vi "曲线对齐-多曲线.vi"() -> ()   [LabVIEW 2015]
uses:
  <vilib>/Utility/miscctls.llb/LVCursorListTypeDef.ctl
  <vilib>/gmath/NI_Gmath.lvlib
panel:
  in  "参考曲线":u16(ring) items=["数据1", "数据2"]
  in  "编辑曲线":u16(ring) items=["数据1", "数据2"]
  in  "重采样间隔":dbl=0.1 min=1e-06 format="%.3fs"
  in  "取消修改":bool
  in  "当前编辑曲线":T1
  in  "确认修改":bool
  in  "功能选择":T2
  in  "加载数据":bool
  out "曲线对齐":cluster{"理论时间":dbl[], "力":dbl[]}[](graph)
  in  "测量曲线路径":path=path "D:/曲线处理/数据源.csv" caption="数据源"
  in  "Enqueue Element":bool caption="元素入队列"
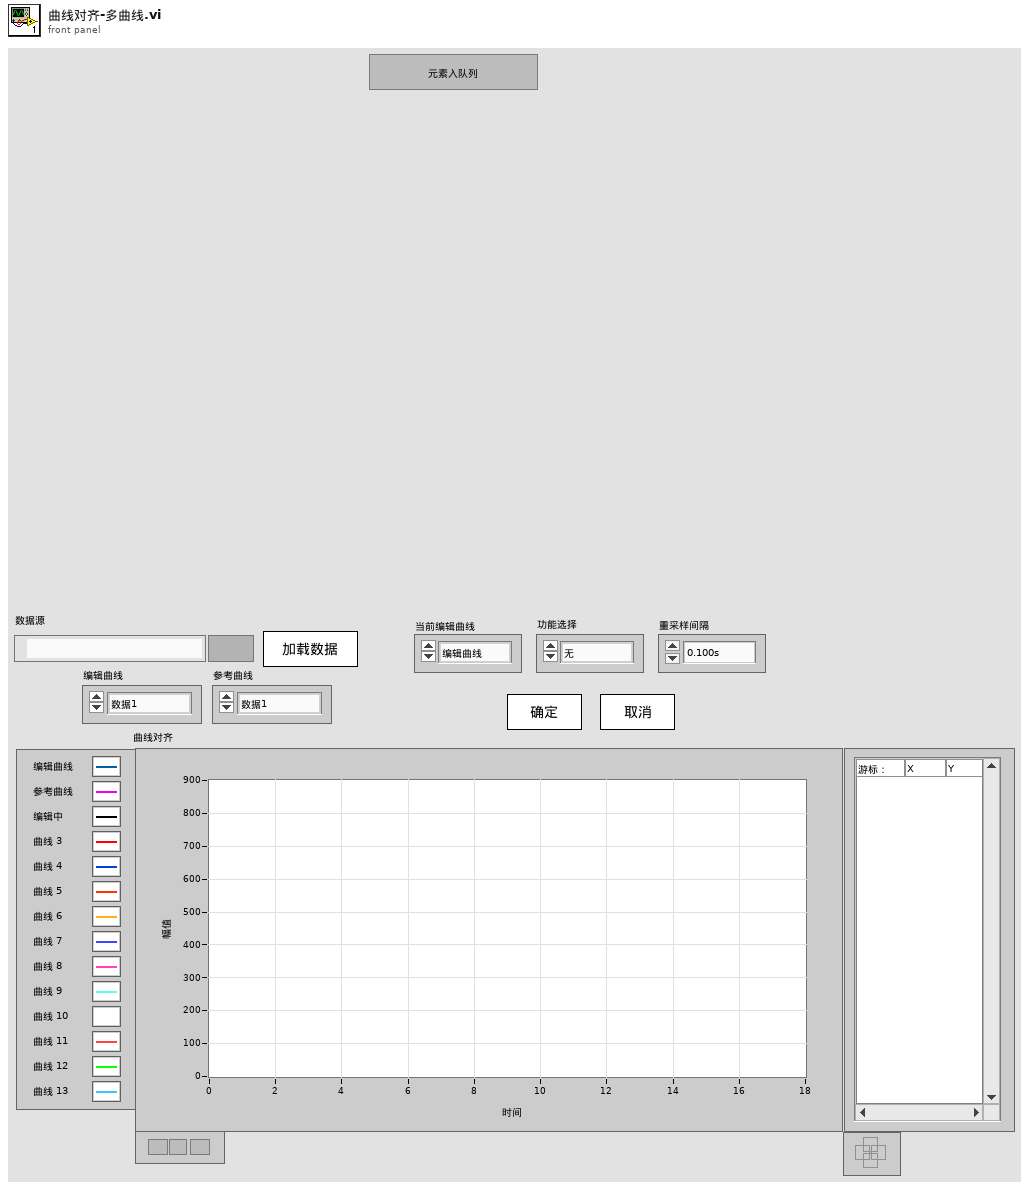
[diagram p1: front panel]
types:
  T1 = typedef "曲线选择.ctl" = enum16{"编辑曲线", "参考曲线"}
  T2 = typedef "功能选择.ctl" = enum16{"无", "缩放曲线", "剪裁曲线", "对齐曲线", "初始值置0", "重采样", "曲线平滑"}
  T3 = typedef "曲线定义.ctl" = enum16{"编辑曲线", "参考曲线", "编辑中曲线"}
  T4 = typedef "LVCursorListTypeDef.ctl" = cluster{"Name":string, "Color":u32, "Style":u8, "Point Style":u8, "Name Visible":bool, "Allow Drag":bool, "Cursor Mode":u32, "Plot":i32, "Index":i32, "Position":cluster{"X":dbl, "Y":dbl}, "X Scale":u32, "Y Scale":u32, "Watch Plots":i32[], "Watch All Plots":bool, "Plot Area":i32, "Label Offset":cluster{"X":dbl, "Y":dbl}}[]
  T5 = cluster{"Name":string, "Color":u32, "Style":u8, "Point Style":u8, "Name Visible":bool, "Allow Drag":bool, "Cursor Mode":u32, "Plot":i32, "Index":i32, "Position":cluster{"X":dbl, "Y":dbl}, "X Scale":u32, "Y Scale":u32, "Watch Plots":i32[], "Watch All Plots":bool, "Plot Area":i32, "Label Offset":cluster{"X":dbl, "Y":dbl}}
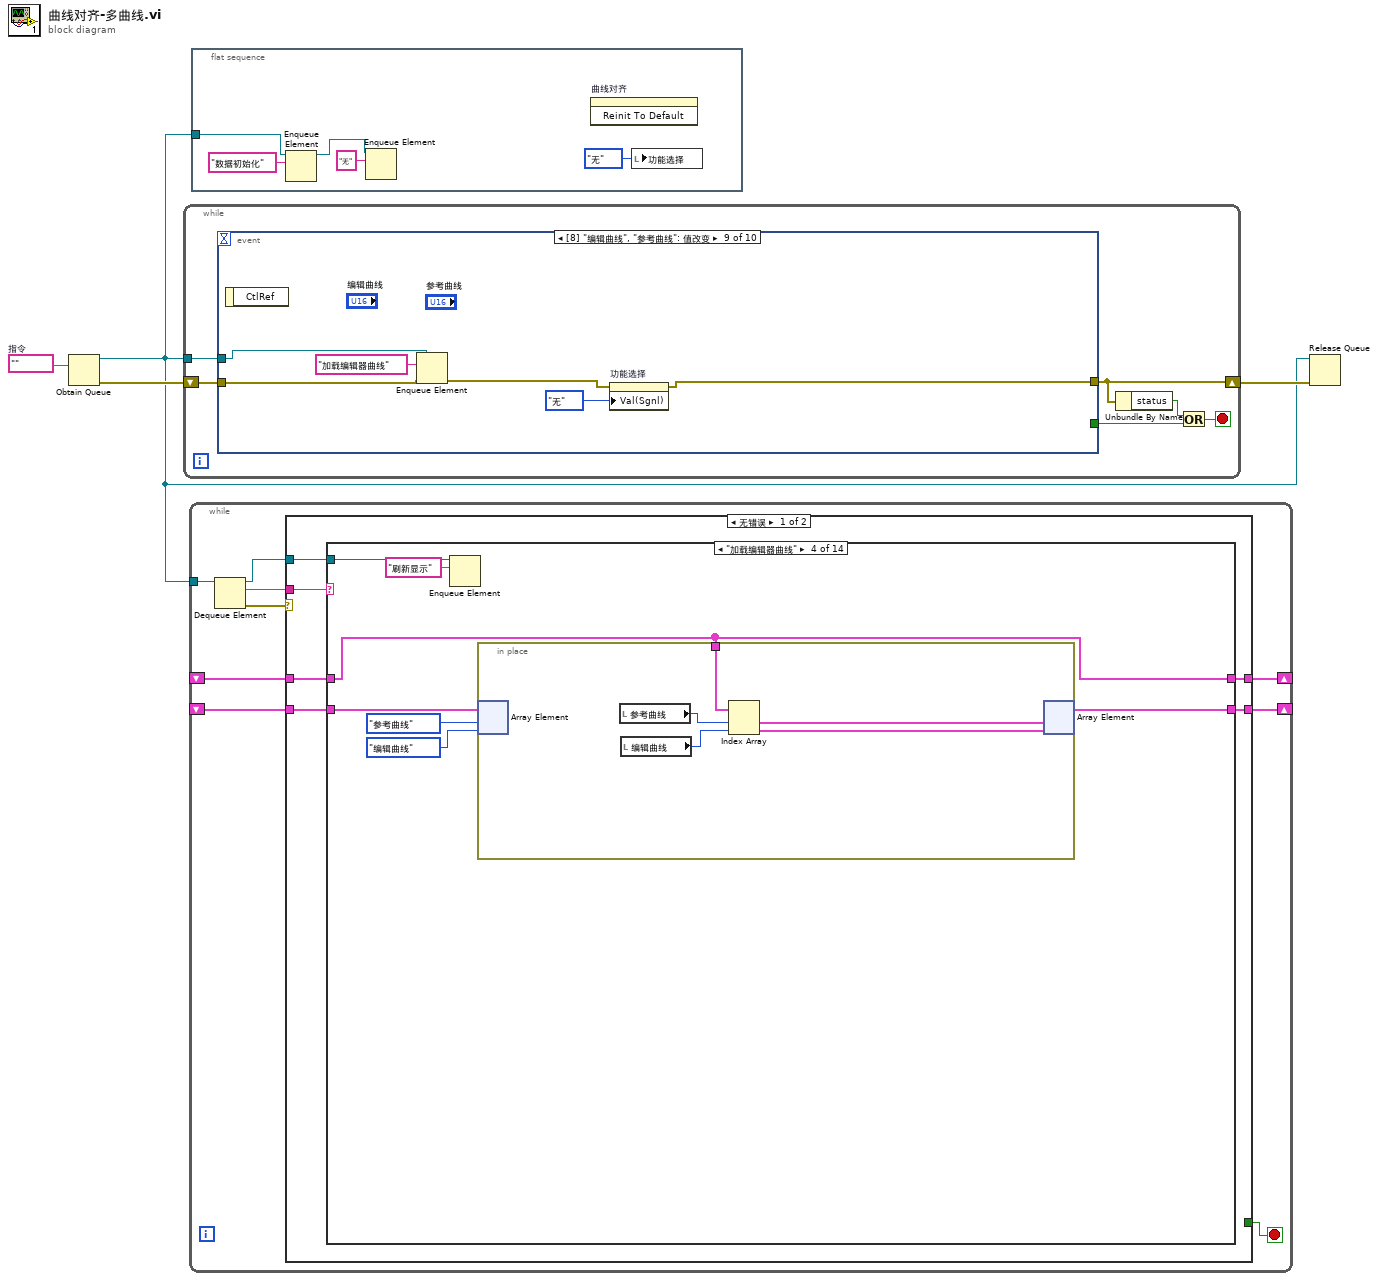
[diagram p0: block diagram]
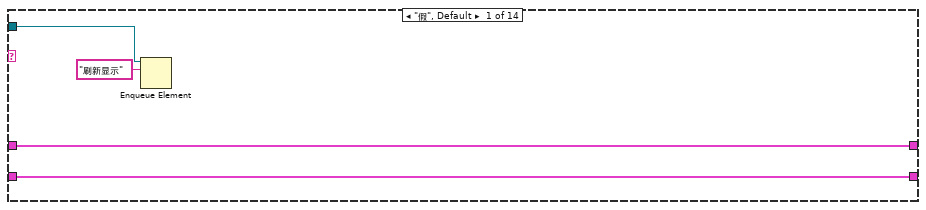
[diagram p2: hidden frame]
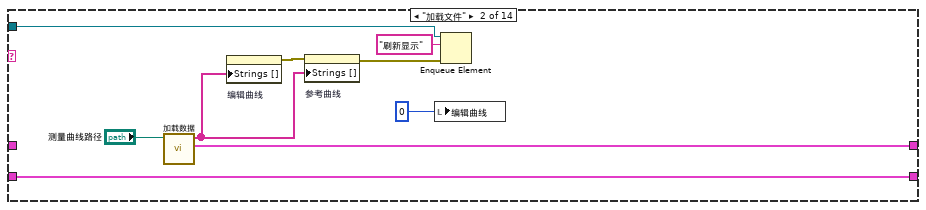
[diagram p3: hidden frame]
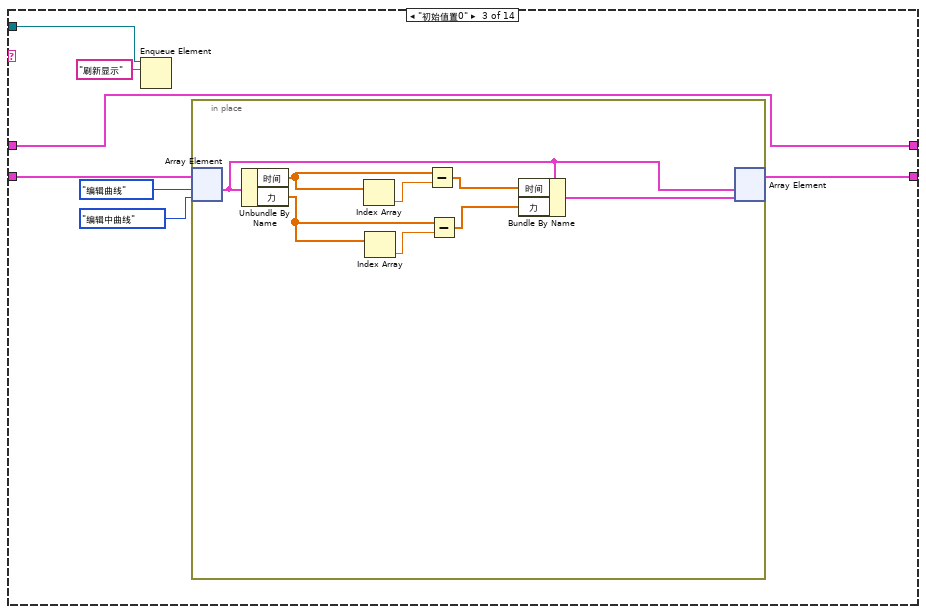
[diagram p4: hidden frame]
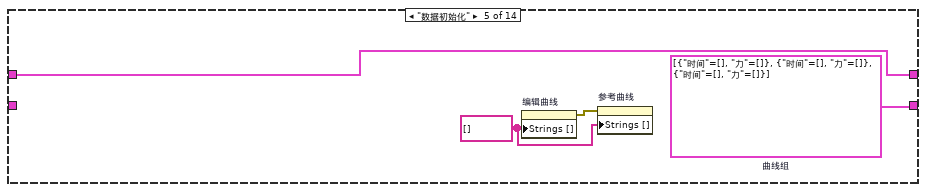
[diagram p5: hidden frame]
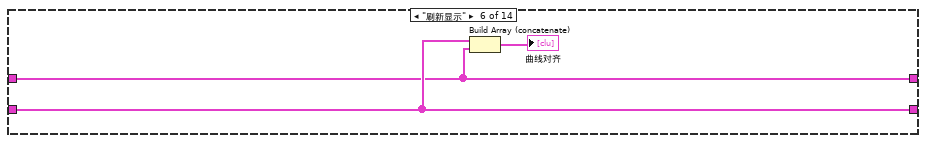
[diagram p6: hidden frame]
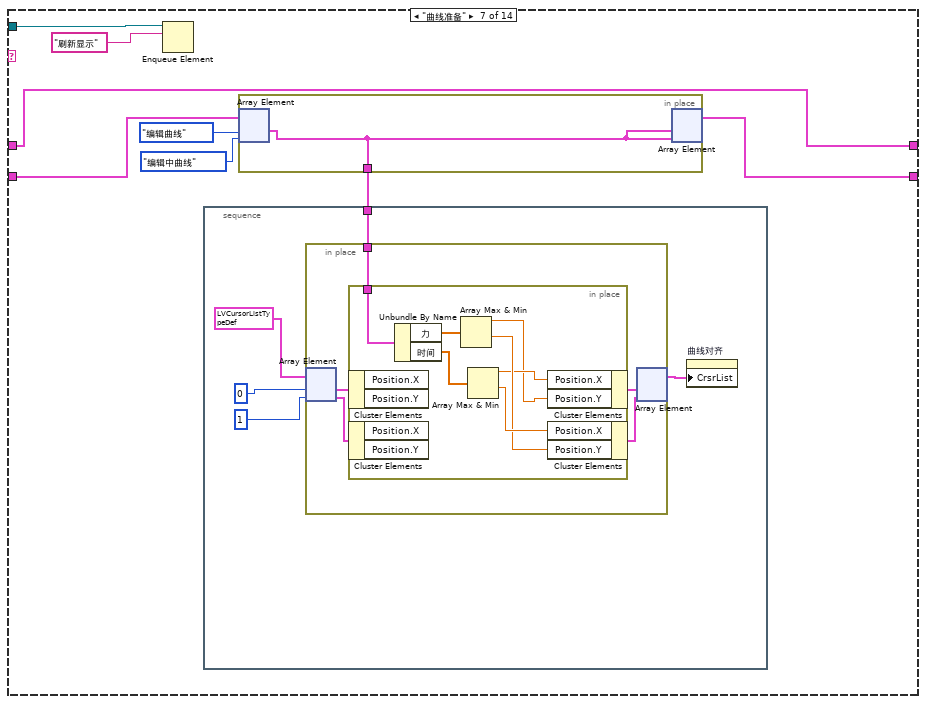
[diagram p7: hidden frame]
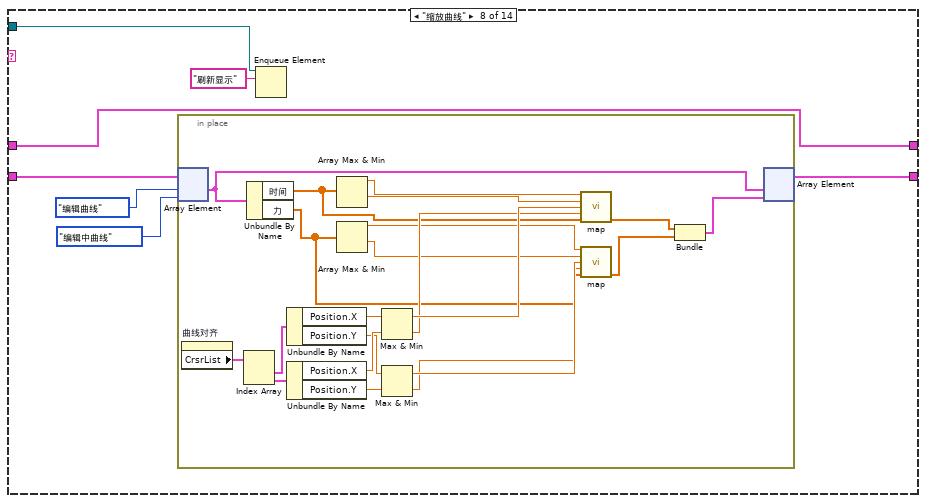
[diagram p8: hidden frame]
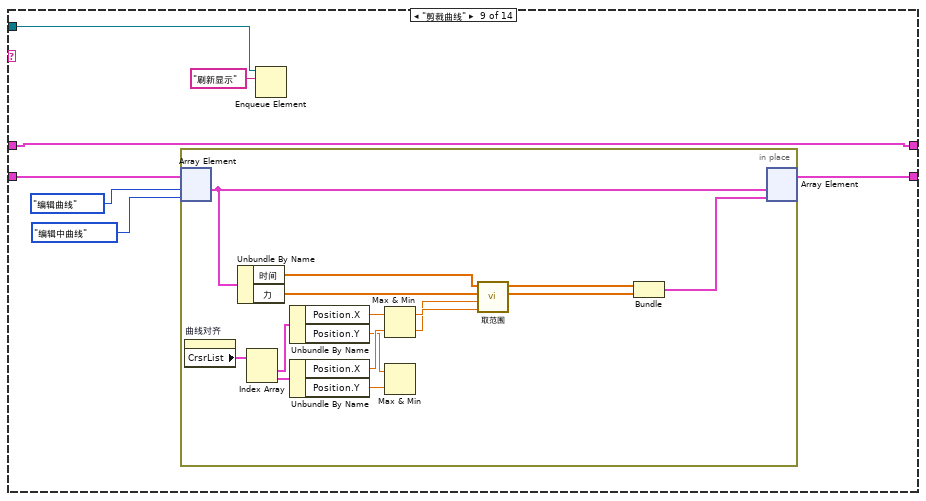
[diagram p9: hidden frame]
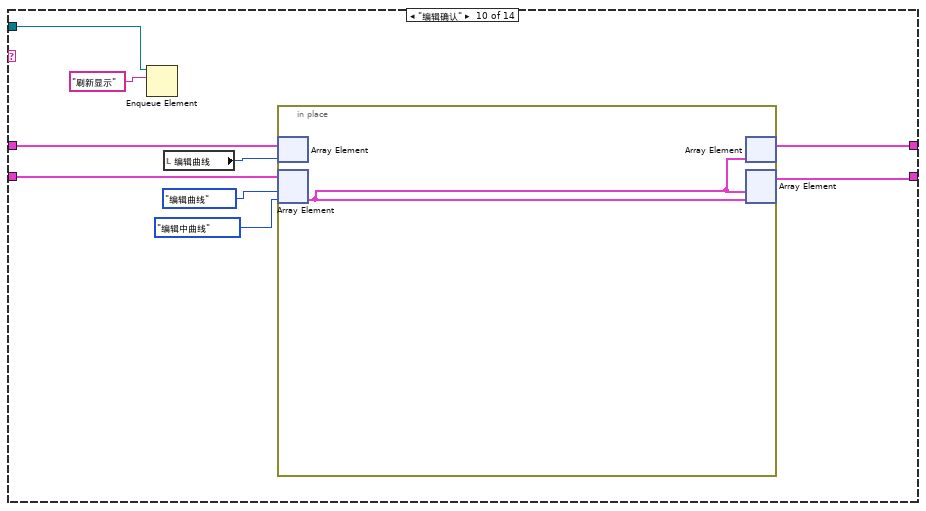
[diagram p10: hidden frame]
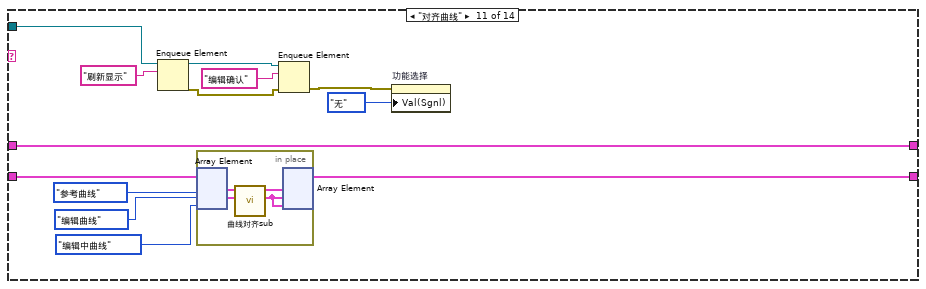
[diagram p11: hidden frame]
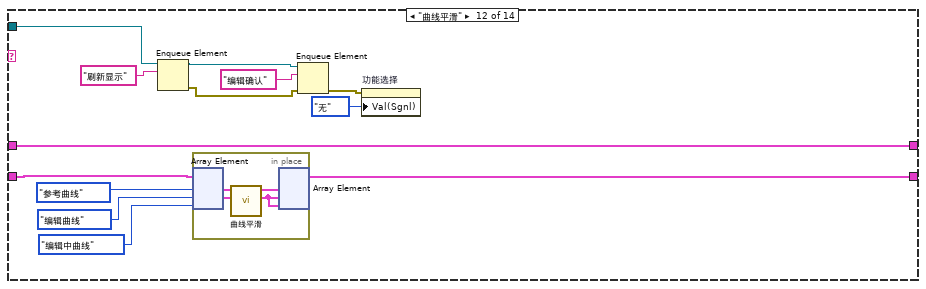
[diagram p12: hidden frame]
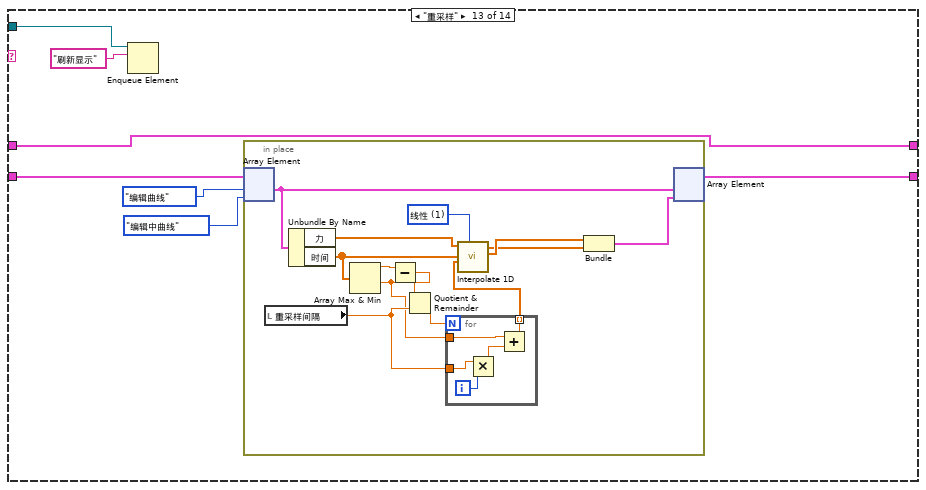
[diagram p13: hidden frame]
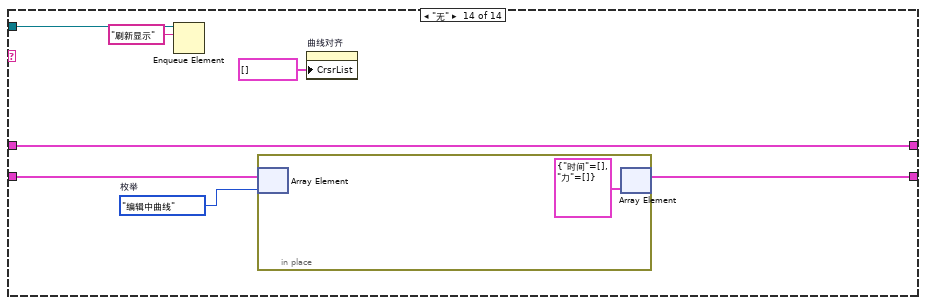
[diagram p14: hidden frame]
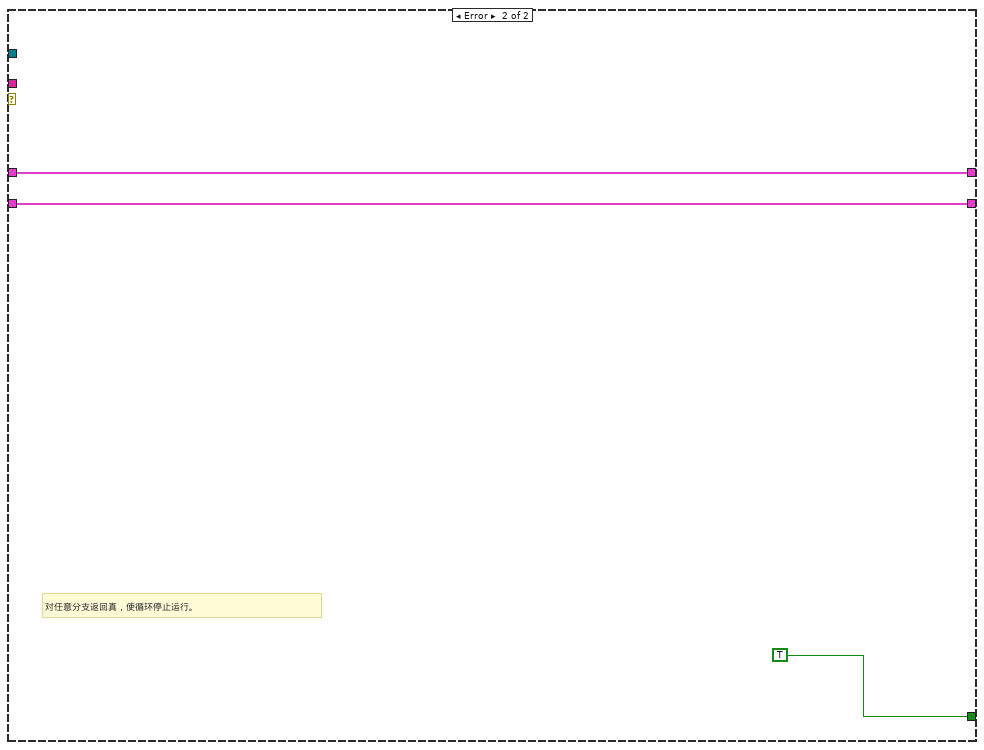
[diagram p15: hidden frame]
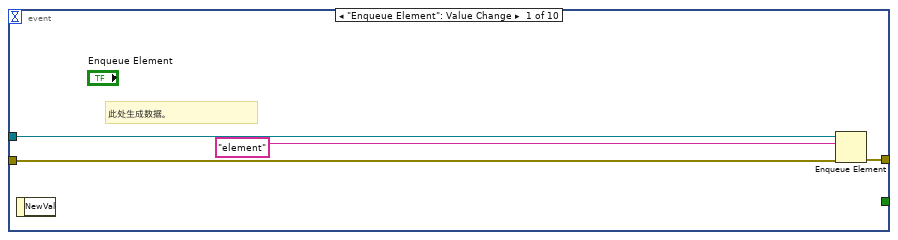
[diagram p16: hidden frame]
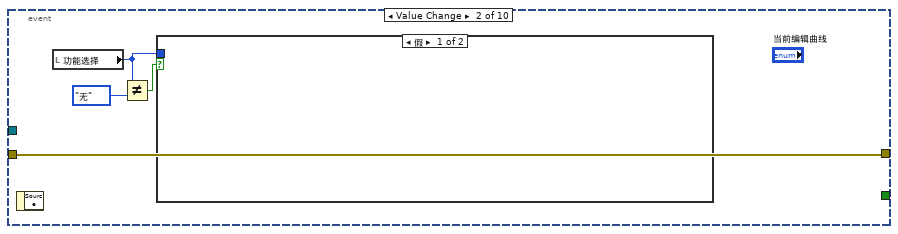
[diagram p17: hidden frame]
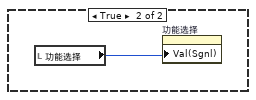
[diagram p18: hidden frame]
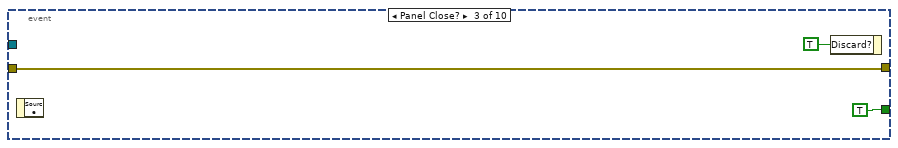
[diagram p19: hidden frame]
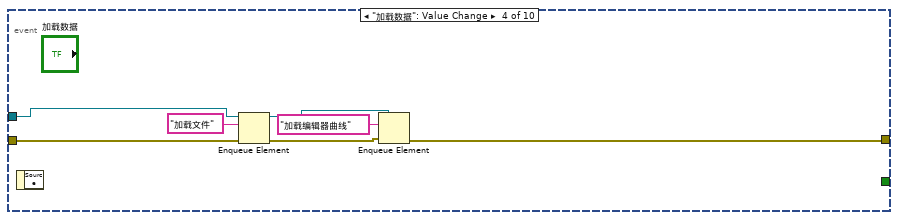
[diagram p20: hidden frame]
diagram:
  w4 = ""  # 指令
  n1 = Obtain Queue(element data type=w4) -> (queue out=w1:refnum<queue>, error out=w2:errorcluster)  [unwired: 4 in, 1 out]
  n2 = while {
    shift-right: [w6] -> w3
    shift-left: w2 -> [w9]
    tunnel: w1 -> [w10]
    stop <- w7 stop-if-true
    n3 = event shown="[8] \"编辑曲线\", \"参考曲线\": 值改变" {
      selector: _ -> [_ _ _ _ _ _ _ _ _ _]
      dyn-events: _ -> [_ _ _ _ _ _ _ _ _ _]
      timeout: _ -> [_ _ _ _ _ _ _ _ _ _]
      tunnel: w10 -> [w14 _ _ w27 w33 _ w43 w49 w70 w72]
      tunnel: w9 -> [w13 w18 w22 w26 w34 w38 w44 w51 w69 w74]
      tunnel: [w12 w18 w22 w23 w34 w37 w44 w51 w66 w74] -> w6
      tunnel: [_ _ TRUE ("stop") _ _ _ _ _ _ _] -> w8
      event "Enqueue Element": Value Change {
        # "此处生成数据。"
        n4 = event-data() -> ()  [unwired: 1 in, 1 out]
        n5 = Enqueue Element(queue=w14, element="element", error in (no error)=w13) -> (error out=w12:errorcluster)  [unwired: 1 in, 2 out]
      }
      event Value Change {
        n6 = event-data() -> ()  [unwired: 1 in, 1 out]
        n7 = local read "功能选择"() -> (w15:T2)
        n8 = Not Equal?(x=w15, y=功能选择."无") -> (x != y?=w17:bool)
        n9 = case shown="假" w17 {
          tunnel: w15 -> [_ _]
          frame False {
          }
          frame True {
            n10 = local read "功能选择"() -> (w19:T2)
            n11 = property on="功能选择" class="Enum (严格)"("Val(Sgnl)"=w19) -> ()  [unwired: 2 in, 2 out]
          }
        }
      }
      event Panel Close? {
        n12 = event-data() -> ()  [unwired: 1 in, 1 out]
        n13 = event-data("Discard?"=TRUE ("放弃？")) -> ()  [unwired: 1 in, 1 out]
      }
      event "加载数据": Value Change {
        n14 = event-data() -> ()  [unwired: 1 in, 1 out]
        n15 = Enqueue Element(queue=w27, element="加载文件" ("元素"), error in (no error)=w26) -> (queue out=w24:refnum<queue>, error out=w25:errorcluster)  [unwired: 1 in, 1 out]
        n16 = Enqueue Element(queue=w24, element="加载编辑器曲线" ("元素"), error in (no error)=w25) -> (error out=w23:errorcluster)  [unwired: 1 in, 2 out]
      }
      event "确认修改": Value Change {
        n17 = event-data() -> ()  [unwired: 1 in, 1 out]
        n18 = local read "功能选择"() -> (w32:T2)
        n19 = Not Equal?(x=w32, y=功能选择."无") -> (x != y?=w31:bool)
        n20 = case shown="真" w31 {
          tunnel: w33 -> [_ w35]
          frame False {
          }
          frame True {
            n21 = Enqueue Element(queue=w35, element="编辑确认" ("元素")) -> ()  [unwired: 2 in, 3 out]
          }
        }
      }
      event "取消修改": Value Change {
        n22 = event-data() -> ()  [unwired: 1 in, 1 out]
        n23 = property on="功能选择" class="Enum (严格)"(error in=w38, "Val(Sgnl)"=功能选择."无" ("值(信号)")) -> (error out=w37:errorcluster)  [unwired: 1 in, 1 out]
      }
      event "重采样间隔": Value Change {
        n24 = event-data() -> ()  [unwired: 1 in, 1 out]
        n25 = local read "功能选择"() -> (w41:T2)
        n26 = Equal?(x=w41, y=功能选择."重采样") -> (x = y?=w42:bool)
        n27 = case shown="真" w42 {
          tunnel: w43 -> [_ w45]
          frame False {
          }
          frame True {
            n28 = Enqueue Element(queue=w45, element="重采样" ("元素")) -> ()  [unwired: 2 in, 3 out]
          }
        }
      }
      event Value Change {
        n29 = event-data() -> ("NewVal"=w50:T2)  [unwired: 1 in]
        n30 = Enqueue Element(queue=w49, element="无" ("元素")) -> (queue out=w48:refnum<queue>)  [unwired: 2 in, 2 out]
        n31 = case shown="\"初始值置0\"" w50 {
          tunnel: w48 -> [w52 w55 w56 w58 w60 w63 w64]
          frame "缩放曲线", Default {
            n32 = Enqueue Element(queue=w52, element="曲线准备" ("元素")) -> ()  [unwired: 2 in, 3 out]
          }
          frame "无" {
            n33 = Enqueue Element(queue=w55, element="无" ("元素")) -> ()  [unwired: 2 in, 3 out]
          }
          frame "剪裁曲线" {
            n34 = Enqueue Element(queue=w56, element="曲线准备" ("元素")) -> ()  [unwired: 2 in, 3 out]
          }
          frame "对齐曲线" {
            n35 = Enqueue Element(queue=w58, element="对齐曲线" ("元素")) -> ()  [unwired: 2 in, 3 out]
          }
          frame "初始值置0" {
            n36 = Enqueue Element(queue=w60, element="初始值置0" ("元素")) -> ()  [unwired: 2 in, 3 out]
          }
          frame "重采样" {
            n37 = Enqueue Element(queue=w63, element="重采样" ("元素")) -> ()  [unwired: 2 in, 3 out]
          }
          frame "曲线平滑" {
            n38 = Enqueue Element(queue=w64, element="曲线平滑" ("元素")) -> ()  [unwired: 2 in, 3 out]
          }
        }
      }
      event "编辑曲线", "参考曲线": Value Change {
        n39 = event-data() -> ()  [unwired: 1 in, 1 out]
        n40 = Enqueue Element(queue=w70, element="加载编辑器曲线" ("元素"), error in (no error)=w69) -> (error out=w67:errorcluster)  [unwired: 1 in, 2 out]
        n41 = property on="功能选择" class="Enum (严格)"(error in=w67, "Val(Sgnl)"=功能选择."无" ("功能选择")) -> (error out=w66:errorcluster)  [unwired: 1 in, 1 out]
      }
      event "曲线对齐": Cursor Move {
        n42 = event-data() -> ()  [unwired: 1 in, 8 out]
        n43 = local read "功能选择"() -> (w73:T2)
        n44 = case shown="\"无\", 默认" w73 {
          tunnel: w72 -> [_ w75 w77]
          frame "无", Default {
          }
          frame "缩放曲线" {
            n45 = Enqueue Element(queue=w75, element="缩放曲线" ("元素")) -> ()  [unwired: 2 in, 3 out]
          }
          frame "剪裁曲线" {
            n46 = Enqueue Element(queue=w77, element="剪裁曲线" ("元素")) -> ()  [unwired: 2 in, 3 out]
          }
        }
      }
    }
    n47 = Unbundle By Name(w6) -> ("status"=w5:bool)
    n48 = Or(x=w5, y=w8) -> (x .or. y?=w7:bool)
  }
  n49 = while {
    tunnel: w1 -> [w82]
    shift-right: [w84] -> _
    shift-left: _ -> [w83]
    shift-right: [w80] -> _
    shift-left: _ -> [w79]
    stop <- w85 stop-if-true
    n50 = Dequeue Element(queue=w82) -> (queue out=w81:refnum<queue>, element=w86:string, error out=w87:errorcluster)  [unwired: 2 in, 1 out]
    n51 = case shown="无错误" w87 {
      tunnel: w86 -> [w93 _]
      tunnel: [_ TRUE] -> w85
      tunnel: [w90 w295] -> w84
      tunnel: w83 -> [w92 w295]
      tunnel: w81 -> [w91 _]
      tunnel: [w89 w294] -> w80
      tunnel: w79 -> [w88 w294]
      frame No Error {
        n52 = case shown="\"加载编辑器曲线\"" w93 {
          tunnel: [w95 w104 w111 w125 w137 w140 w144 w170 w198 w222 w236 w252 w264 w287] -> w90
          tunnel: w92 -> [w95 w104 w110 w126 _ w140 w145 w171 w199 w223 w235 w253 w265 w288]
          tunnel: w91 -> [w96 w105 w112 w128 _ _ w147 w172 w200 w224 w238 w255 w266 w290]
          tunnel: [w94 w102 w107 w123 w136 w139 w141 w167 w195 w217 w231 w248 w261 w289] -> w89
          tunnel: w88 -> [w94 _ w107 w123 w136 w139 w141 w167 w195 w218 w231 w248 w261 w289]
          frame "假", Default {
            n53 = Enqueue Element(queue=w96, element="刷新显示" ("元素")) -> ()  [unwired: 2 in, 3 out]
          }
          frame "加载文件" {
            n54 = call "加载数据.vi"("数据路径"="测量曲线路径") -> ("数据"=w102:cluster{dbl[], dbl[]}[], "数据名称"=w100:string[])  [unwired: 9 in]
            n55 = property on="编辑曲线" class="Ring (严格)"("Strings []"=w100) -> (error out=w99:errorcluster)  [unwired: 2 in, 1 out]
            n56 = property on="参考曲线" class="Ring (严格)"(error in=w99, "Strings []"=w100) -> (error out=w98:errorcluster)  [unwired: 1 in, 1 out]
            n57 = local write "编辑曲线"(0) -> ()
            n58 = Enqueue Element(queue=w105, element="刷新显示" ("元素"), error in (no error)=w98) -> ()  [unwired: 1 in, 3 out]
          }
          frame "初始值置0" {
            n59 = Enqueue Element(queue=w112, element="刷新显示" ("元素")) -> ()  [unwired: 2 in, 3 out]
            n60 = in-place {
              n61 = in-place-array #1(w110, 曲线定义."编辑曲线", 曲线定义."编辑中曲线") -> (w115:cluster{"时间":dbl[], "力":dbl[]})  [unwired: 1 out]
              n62 = Unbundle By Name(w115) -> ("时间"=w121:dbl[], "力"=w119:dbl[])
              n63 = Index Array(array=w121) -> (element=w120:dbl)  [unwired: 1 in]
              n64 = Index Array(array=w119) -> (element=w118:dbl)  [unwired: 1 in]
              n65 = Subtract(x=w121, y=w120) -> (x-y=w117:dbl[])
              n66 = Subtract(x=w119, y=w118) -> (x-y=w116:dbl[])
              n67 = Bundle By Name(cluster=w115, "时间"=w117, "力"=w116) -> (w114:cluster{"时间":dbl[], "力":dbl[]})
              n68 = in-place-array #1(w115, w114) -> (w111:cluster{"时间":dbl[], "力":dbl[]}[])  [unwired: 2 out]
            }
          }
          frame "加载编辑器曲线" {
            n69 = Enqueue Element(queue=w128, element="刷新显示" ("元素")) -> ()  [unwired: 2 in, 3 out]
            n70 = in-place {
              in-place-border: w123 -> [w133]
              n71 = in-place-array #2(w126, 曲线定义."参考曲线", 曲线定义."编辑曲线") -> ()  [unwired: 2 out]
              n72 = local read "参考曲线"() -> (w129:u16)
              n73 = local read "编辑曲线"() -> (w130:u16)
              n74 = Index Array(array=w133, index #1=w129, index #2=w130) -> (element #1=w132:cluster{dbl[], dbl[]}, element #2=w131:cluster{dbl[], dbl[]})
              n75 = in-place-array #2(w132, w131) -> (w125:cluster{"时间":dbl[], "力":dbl[]}[])  [unwired: 2 out]
            }
          }
          frame "数据初始化" {
            w135 = string[] [] ("字符串[]")
            w137 = cluster{"时间":dbl[], "力":dbl[]}[] [{"时间"=[], "力"=[]}, {"时间"=[], "力"=[]}, {"时间"=[], "力"=[]}]  # 曲线组
            n76 = property on="编辑曲线" class="Ring (严格)"("Strings []"=w135) -> (error out=w134:errorcluster)  [unwired: 2 in, 1 out]
            n77 = property on="参考曲线" class="Ring (严格)"(error in=w134, "Strings []"=w135) -> ()  [unwired: 1 in, 2 out]
          }
          frame "刷新显示" {
            n78 = Build Array (concatenate)(w140, w139) -> (→"曲线对齐":cluster{"时间":dbl[], "力":dbl[]}[])
          }
          frame "曲线准备" {
            n79 = Enqueue Element(queue=w147, element="刷新显示" ("元素")) -> ()  [unwired: 2 in, 3 out]
            n80 = in-place {
              in-place-border: [w149] -> w146
              n81 = in-place-array #3(w145, 曲线定义."编辑曲线", 曲线定义."编辑中曲线") -> (w149:cluster{"时间":dbl[], "力":dbl[]})  [unwired: 1 out]
              n82 = in-place-array #3(w149, w149) -> (w144:cluster{"时间":dbl[], "力":dbl[]}[])  [unwired: 2 out]
            }
            n83 = stacked-sequence {
              tunnel: w146 -> [w150]
              frame #0 {
                n84 = in-place {
                  in-place-border: w150 -> [w155]
                  n85 = in-place-array #4(T4 [{"Name"="游标0", "Color"=16711680, "Style"=8, "Point Style"=13, "Name Visible"=FALSE, "Allow Drag"=TRUE, "Cursor Mode"=0, "Plot"=0, "Index"=0, "Position"={"X"=24.900169204737733, "Y"=876.3513513513514}, "X Scale"=0, "Y Scale"=0, "Watch Plots"=[], "Watch All Plots"=FALSE, "Plot Area"=0, "Label Offset"={"X"=0.0, "Y"=67.56756756756761}}, {"Name"="游标1", "Color"=16860, "Style"=8, "Point Style"=13, "Name Visible"=FALSE, "Allow Drag"=TRUE, "Cursor Mode"=0, "Plot"=0, "Index"=0, "Position"={"X"=-2.199661590524536, "Y"=1.3513513513513553}, "X Scale"=0, "Y Scale"=0, "Watch Plots"=[], "Watch All Plots"=FALSE, "Plot Area"=0, "Label Offset"={"X"=8.881784197001252e-16, "Y"=67.56756756756756}}] ("游标列表"), 0, 1) -> (w159:T5, w158:T5)
                  n86 = in-place {
                    in-place-border: w155 -> [w162]
                    n87 = in-place-cluster #5(w159) -> ()  [unwired: 2 out]
                    n88 = in-place-cluster #6(w158) -> ()  [unwired: 2 out]
                    n89 = Unbundle By Name(w162) -> ("力"=w161:dbl[], "时间"=w160:dbl[])
                    n90 = Array Max & Min(array=w161) -> (max value=w163:dbl, min value=w165:dbl)  [unwired: 2 out]
                    n91 = Array Max & Min(array=w160) -> (max value=w164:dbl, min value=w166:dbl)  [unwired: 2 out]
                    n92 = in-place-cluster #5("Position.X"=w164, "Position.Y"=w163) -> (w157:T5)
                    n93 = in-place-cluster #6("Position.X"=w166, "Position.Y"=w165) -> (w156:T5)
                  }
                  n94 = in-place-array #4(w157, w156) -> (w151:T4)  [unwired: 2 out]
                }
                n95 = property on="曲线对齐" class="XYGraph (严格)"("CrsrList"=w151) -> ()  [unwired: 2 in, 2 out]
              }
            }
          }
          frame "缩放曲线" {
            n96 = in-place {
              n97 = in-place-array #7(w171, 曲线定义."编辑曲线", 曲线定义."编辑中曲线") -> (w176:cluster{"时间":dbl[], "力":dbl[]})  [unwired: 1 out]
              n98 = property on="曲线对齐" class="XYGraph (严格)"() -> ("CrsrList"=w194:T4)  [unwired: 2 in, 2 out]
              n99 = Index Array(array=w194) -> (element #1=w193:T5, element #2=w192:T5)  [unwired: 2 in]
              n100 = Unbundle By Name(w176) -> ("时间"=w175:dbl[], "力"=w174:dbl[])
              n101 = Unbundle By Name(w193) -> ("Position.X"=w191:dbl, "Position.Y"=w189:dbl)
              n102 = Unbundle By Name(w192) -> ("Position.X"=w190:dbl, "Position.Y"=w188:dbl)
              n103 = Array Max & Min(array=w175) -> (max value=w187:dbl, min value=w186:dbl)  [unwired: 2 out]
              n104 = Array Max & Min(array=w174) -> (max value=w183:dbl, min value=w182:dbl)  [unwired: 2 out]
              n105 = Max & Min(x=w191, y=w190) -> (max(x,y)=w185:dbl, min(x,y)=w184:dbl)
              n106 = Max & Min(x=w189, y=w188) -> (max(x,y)=w181:dbl, min(x,y)=w180:dbl)
              n107 = call "map.vi"("inmax"=w187, "inmin"=w186, "outmax"=w185, "outmin"=w184, "in"=w175) -> ("out"=w179:dbl[])  [unwired: 10 in]
              n108 = call "map.vi"("inmax"=w183, "inmin"=w182, "outmax"=w181, "outmin"=w180, "in"=w174) -> ("out"=w178:dbl[])  [unwired: 10 in]
              n109 = Bundle("out"=w179, "out"=w178) -> (w177:cluster{"out":dbl[], "out":dbl[]})  [unwired: 1 in]
              n110 = in-place-array #7(w176, w177) -> (w170:cluster{"时间":dbl[], "力":dbl[]}[])  [unwired: 2 out]
            }
            n111 = Enqueue Element(queue=w172, element="刷新显示" ("元素")) -> ()  [unwired: 2 in, 3 out]
          }
          frame "剪裁曲线" {
            n112 = in-place {
              n113 = in-place-array #8(w199, 曲线定义."编辑曲线", 曲线定义."编辑中曲线") -> (w209:cluster{"时间":dbl[], "力":dbl[]})  [unwired: 1 out]
              n114 = property on="曲线对齐" class="XYGraph (严格)"() -> ("CrsrList"=w216:T4)  [unwired: 2 in, 2 out]
              n115 = Unbundle By Name(w209) -> ("时间"=w206:dbl[], "力"=w205:dbl[])
              n116 = Index Array(array=w216) -> (element #1=w215:T5, element #2=w214:T5)  [unwired: 2 in]
              n117 = Unbundle By Name(w215) -> ("Position.X"=w213:dbl, "Position.Y"=w211:dbl)
              n118 = Unbundle By Name(w214) -> ("Position.X"=w212:dbl, "Position.Y"=w210:dbl)
              n119 = Max & Min(x=w213, y=w212) -> (max(x,y)=w208:dbl, min(x,y)=w207:dbl)
              n120 = Max & Min(x=w211, y=w210) -> ()  [unwired: 2 out]
              n121 = call "取范围.vi"("max"=w208, "min"=w207, "y"=w205, "x"=w206) -> ("y"=w203:dbl[], "x"=w204:dbl[])  [unwired: 6 in]
              n122 = Bundle("x"=w204, "y"=w203) -> (w202:cluster{"x":dbl[], "y":dbl[]})  [unwired: 1 in]
              n123 = in-place-array #8(w209, w202) -> (w198:cluster{"时间":dbl[], "力":dbl[]}[])  [unwired: 2 out]
            }
            n124 = Enqueue Element(queue=w200, element="刷新显示" ("元素")) -> ()  [unwired: 2 in, 3 out]
          }
          frame "编辑确认" {
            n125 = Enqueue Element(queue=w224, element="刷新显示" ("元素")) -> ()  [unwired: 2 in, 3 out]
            n126 = local read "编辑曲线"() -> (w219:u16)
            n127 = in-place {
              n128 = in-place-array #9(w218, w219) -> ()  [unwired: 1 out]
              n129 = in-place-array #10(w223, 曲线定义."编辑曲线", 曲线定义."编辑中曲线") -> (w226:cluster{"时间":dbl[], "力":dbl[]})  [unwired: 1 out]
              n130 = in-place-array #9(w226) -> (w217:cluster{dbl[], dbl[]}[])  [unwired: 1 out]
              n131 = in-place-array #10(w226, w226) -> (w222:cluster{"时间":dbl[], "力":dbl[]}[])  [unwired: 2 out]
            }
          }
          frame "对齐曲线" {
            n132 = Enqueue Element(queue=w238, element="刷新显示" ("元素")) -> (queue out=w229:refnum<queue>, error out=w227:errorcluster)  [unwired: 2 in, 1 out]
            n133 = in-place {
              n134 = in-place-array #11(w235, 曲线定义."参考曲线", 曲线定义."编辑曲线", 曲线定义."编辑中曲线") -> (w243:cluster{"时间":dbl[], "力":dbl[]}, w242:cluster{"时间":dbl[], "力":dbl[]})  [unwired: 1 out]
              n135 = call "曲线对齐sub.vi"("测量"=w242, "理论"=w243) -> ("实测"=w240:cluster{dbl[], dbl[]}, "理论"=w241:cluster{dbl[], dbl[]})  [unwired: 8 in]
              n136 = in-place-array #11(w241, w240, w240) -> (w236:cluster{"时间":dbl[], "力":dbl[]}[])  [unwired: 3 out]
            }
            n137 = Enqueue Element(queue=w229, element="编辑确认" ("元素"), error in (no error)=w227) -> (error out=w228:errorcluster)  [unwired: 1 in, 2 out]
            n138 = property on="功能选择" class="Enum (严格)"(error in=w228, "Val(Sgnl)"=功能选择."无" ("功能选择")) -> ()  [unwired: 1 in, 2 out]
          }
          frame "曲线平滑" {
            n139 = Enqueue Element(queue=w255, element="刷新显示" ("元素")) -> (queue out=w246:refnum<queue>, error out=w245:errorcluster)  [unwired: 2 in, 1 out]
            n140 = in-place {
              n141 = in-place-array #12(w253, 曲线定义."参考曲线", 曲线定义."编辑曲线", 曲线定义."编辑中曲线") -> (w260:cluster{"时间":dbl[], "力":dbl[]}, w259:cluster{"时间":dbl[], "力":dbl[]})  [unwired: 1 out]
              n142 = call "曲线平滑.vi"("测量"=w259, "理论"=w260) -> ("实测"=w257:cluster{dbl[], dbl[]}, "理论"=w258:cluster{dbl[], dbl[]})  [unwired: 8 in]
              n143 = in-place-array #12(w258, w257, w257) -> (w252:cluster{"时间":dbl[], "力":dbl[]}[])  [unwired: 3 out]
            }
            n144 = Enqueue Element(queue=w246, element="编辑确认" ("元素"), error in (no error)=w245) -> (error out=w244:errorcluster)  [unwired: 1 in, 2 out]
            n145 = property on="功能选择" class="Enum (严格)"(error in=w244, "Val(Sgnl)"=功能选择."无" ("功能选择")) -> ()  [unwired: 1 in, 2 out]
          }
          frame "重采样" {
            n146 = Enqueue Element(queue=w266, element="刷新显示" ("元素")) -> ()  [unwired: 2 in, 3 out]
            n147 = in-place {
              w280 = 1 items=["最近", "线性", "样条", "cubic Hermite", "拉格朗日"] ("method")
              n148 = in-place-array #13(w265, 曲线定义."编辑曲线", 曲线定义."编辑中曲线") -> (w274:cluster{"时间":dbl[], "力":dbl[]})  [unwired: 1 out]
              n149 = local read "重采样间隔"() -> (w272:dbl)
              n150 = Unbundle By Name(w274) -> ("力"=w279:dbl[], "时间"=w278:dbl[])
              n151 = Array Max & Min(array=w278) -> (max value=w271:dbl, min value=w269:dbl)  [unwired: 2 out]
              n152 = Subtract(x=w271, y=w269) -> (x-y=w270:dbl)
              n153 = Quotient & Remainder(x=w270, y=w272) -> (floor(x/y)=w273:dbl)  [unwired: 1 out]
              n154 = for {
                N: w273 -> [_]
                tunnel: w272 -> [w284]
                tunnel: w269 -> [w282]
                tunnel: [w281] -> w268 mode=indexing
                i -> [w285]
                n155 = Multiply(x=w284, y=w285) -> (x*y=w283:dbl)
                n156 = Add(x=w282, y=w283) -> (x+y=w281:dbl)
              }
              n157 = call <vilib>:"Interpolate 1D.vi"("method"=w280, "xi"=w268, "X"=w278, "Y"=w279) -> ("xi used"=w277:dbl[], "yi"=w276:dbl[])  [unwired: 5 in, 1 out]
              n158 = Bundle("xi used"=w277, "yi"=w276) -> (w275:cluster{"xi used":dbl[], "yi":dbl[]})  [unwired: 1 in]
              n159 = in-place-array #13(w274, w275) -> (w264:cluster{"时间":dbl[], "力":dbl[]}[])  [unwired: 2 out]
            }
          }
          frame "无" {
            w286 = 曲线定义."编辑中曲线"  # 枚举
            n160 = Enqueue Element(queue=w290, element="刷新显示" ("元素")) -> ()  [unwired: 2 in, 3 out]
            n161 = in-place {
              n162 = in-place-array #14(w288, w286) -> ()  [unwired: 1 out]
              n163 = in-place-array #14(cluster{"时间":dbl[], "力":dbl[]} {"时间"=[], "力"=[]} ("元素")) -> (w287:cluster{"时间":dbl[], "力":dbl[]}[])  [unwired: 1 out]
            }
            n164 = property on="曲线对齐" class="XYGraph (严格)"("CrsrList"=T4 [] ("游标列表")) -> ()  [unwired: 2 in, 2 out]
          }
        }
      }
      frame Error {
        # "对任意分支返回真，使循环停止运行。"
      }
    }
  }
  n165 = flat-sequence {
    tunnel: w1 -> [w300]
    frame #0 {
      n166 = Enqueue Element(queue=w300, element="数据初始化" ("元素")) -> (queue out=w298:refnum<queue>)  [unwired: 2 in, 2 out]
      n167 = Enqueue Element(queue=w298, element="无" ("元素")) -> ()  [unwired: 2 in, 3 out]
      n168 = invoke on="曲线对齐" class="XYGraph (严格)" method="Reinit To Default"() -> ()  [unwired: 3 in, 3 out]
      n169 = local write "功能选择"(功能选择."无" ("功能选择")) -> ()
    }
  }
  n170 = Release Queue(queue=w1, error in (no error)=w3) -> ()  [unwired: 1 in, 3 out]
